vi "get_prod_name.vi"(8 "error in (no error)":errorcluster, 11 "Resources in":refnum<k20>[](array[refnum])) -> (0 "error out":errorcluster, 2 "SerialNum":string[](array[string]), 3 "ProdName":string[](array[string]))   [LabVIEW 2015]
uses:
  <resource>/objmgr/nisysapi.rc
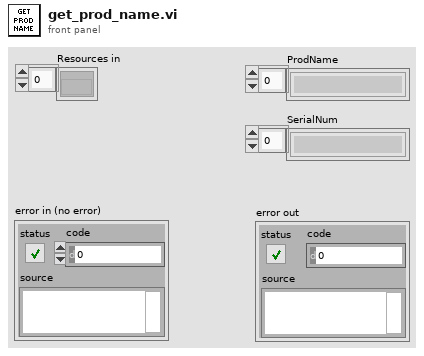
[diagram p1: front panel]
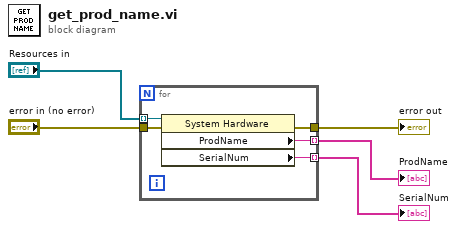
[diagram p0: block diagram]
diagram:
  n1 = for {
    tunnel: "Resources in" -> [w10] mode=indexing
    tunnel: [w9] -> w5 mode=indexing
    tunnel: [w8] -> w4
    tunnel: "error in (no error)" -> [w7]
    tunnel: [w6] -> w1 mode=indexing
    n2 = property class="System Hardware"(reference=w10, error in=w7) -> (error out=w8:errorcluster, "ProdName"=w9:string, "SerialNum"=w6:string)  [unwired: 1 out]
  }
  "ProdName" <- w5
  "error out" <- w4
  "SerialNum" <- w1
